vi "In_Bounds2.vi"(9 "Angle in 3":dbl, 10 "Angle in 2":dbl, 11 "Angle in":dbl) -> (1 "angle 3":dbl, 2 "angle 1":dbl, 3 "angle 2":dbl)   [LabVIEW 2024]
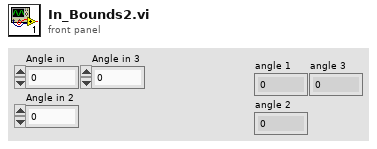
[diagram p1: front panel]
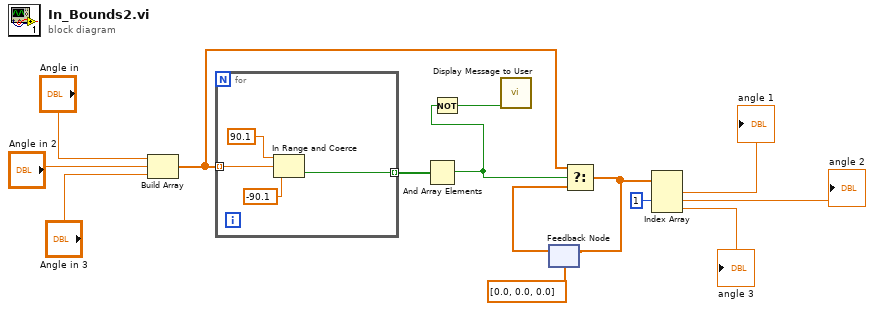
[diagram p0: block diagram]
diagram:
  n1 = Build Array "Build Array"("Angle in", "Angle in 2", "Angle in 3") -> (w10:dbl[])
  n2 = for {
    tunnel: w10 -> [w16] mode=indexing
    tunnel: [w15] -> w11 mode=indexing
    n3 = In Range and Coerce(upper limit=90.1, x=w16, lower limit=-90.1) -> (In Range?=w15:bool)  [unwired: 1 out]
  }
  n4 = And Array Elements(Boolean array=w11) -> (logical AND=w2:bool)
  n5 = Not(x=w2) -> (.not. x?=w3:bool)
  n6 = call "Display Message to User"("Enable"=w3) -> ()  [unwired: 9 in, 2 out]
  n7 = feedback #1(dbl[] [0.0, 0.0, 0.0]) -> (w9:dbl[])
  n8 = Select(t=w10, s=w2, f=w9) -> (s? t:f=w7:dbl[])
  n9 = feedback-in #1(w7) -> ()
  n10 = Index Array "Index Array"(array=w7, index #2=1 ("index")) -> (element #1=→"angle 1":dbl, element #2=→"angle 2":dbl, element #3=→"angle 3":dbl)  [unwired: 2 in]
